vi "Send Message.vi"(8 "error in":errorcluster, 10 "IMessage":refnum<class "IMessage.lvclass">, 11 "ICommunicate in":refnum<class "ICommunicate.lvclass">) -> (0 "error out":errorcluster, 3 "ICommunicate out":refnum<class "ICommunicate.lvclass">)   [LabVIEW 2019, in "ICommunicate.lvclass"]
uses:
  ICommunicate.lvclass
  IMessage/IMessage.lvclass
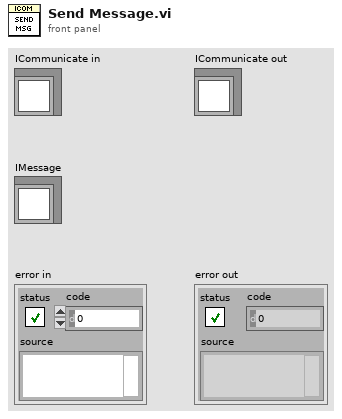
[diagram p1: front panel]
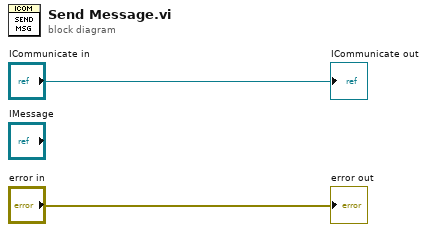
[diagram p0: block diagram]
diagram:
  "error out" <- "error in"
  "ICommunicate out" <- "ICommunicate in"
